vi "Material-Laser-ChangeSamplingRate.vi"(8 "error in (no error)":errorcluster, 11 "Material-RunTest in":refnum<class "Material-RunTest.lvclass">) -> (0 "error out":errorcluster, 2 "Rate updated?":bool, 3 "Material-RunTest out":refnum<class "Material-RunTest.lvclass">)   [LabVIEW 2013, in "Material-RunTest.lvclass"]
uses:
  Material-RunTest.lvclass
  Material-RunTest.lvclass/Material-RunTest.ctl
  <instrlib>/Keyence LK-G5000/Public/enum/LKIF_SamplingRate.ctl
  <instrlib>/Keyence LK-G5000/Keyence LK-G5000.lvlib
  <vilib>/addons/_LabVIEW Style Book/Utilities/Style Book Utilities.lvlib
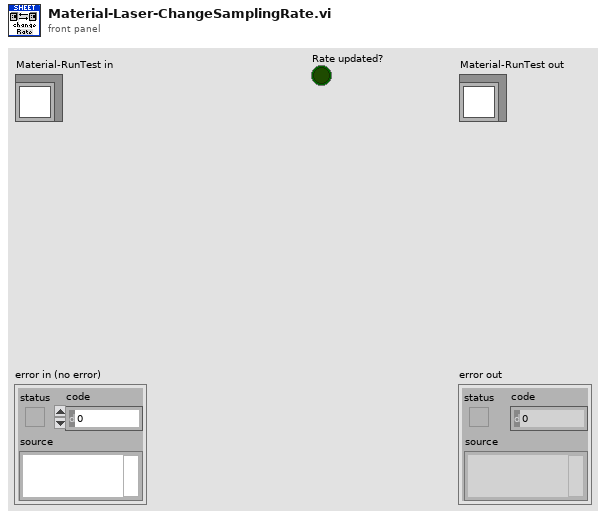
[diagram p1: front panel]
types:
  T1 = typedef "Keyence LK-G5000.lvlib/LKIF_SamplingRate.ctl" = enum16{"2.55uSEC", "5uSEC", "10uSEC", "20uSEC", "50uSEC", "100uSEC", "200uSEC", "500uSEC", "1mSEC"}
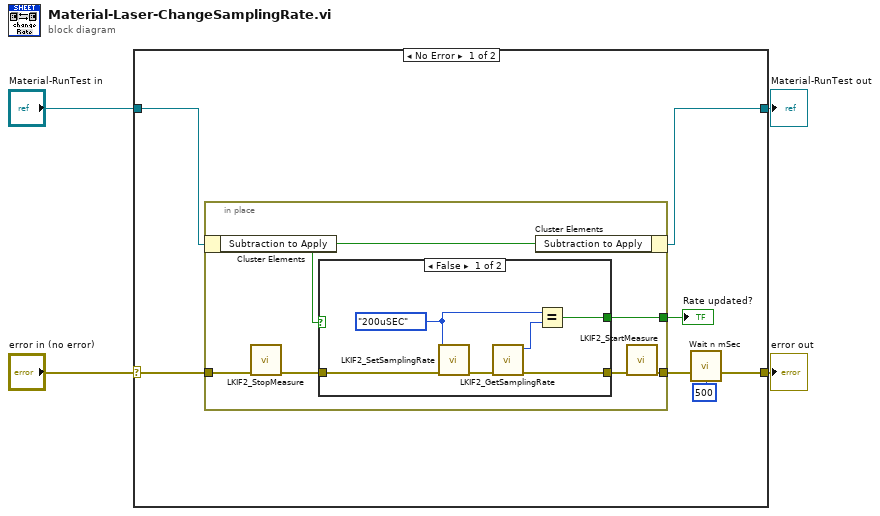
[diagram p0: block diagram]
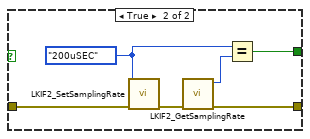
[diagram p2: hidden frame]
diagram:
  n1 = case shown="No Error" "error in (no error)" {
    selector: "error in (no error)" -> [w10 w31]
    tunnel: [w6 w31] -> w3
    tunnel: [w9 w30] -> w1
    tunnel: "Material-RunTest in" -> [w11 w30]
    frame No Error {
      n2 = in-place {
        in-place-border: w10 -> [w17]
        in-place-border: [w14] -> w7
        in-place-border: [w12] -> w8
        n3 = in-place-cluster #1(w11) -> ("Subtraction to Apply"=w13:bool)
        n4 = call <instrlib>:"LKIF2_StopMeasure.vi"("error in (no error)"=w17) -> ("error out"=w16:errorcluster)  [unwired: 10 in]
        n5 = case shown="False" w13 {
          tunnel: w16 -> [w23 w29]
          tunnel: [w21 w26] -> w15
          tunnel: [w18 w24] -> w12
          frame False {
            w20 = LKIF_SamplingRate."200uSEC" ("Sampling Rate")
            n6 = call <instrlib>:"LKIF2_SetSamplingRate.vi"("error in (no error)"=w23, "Sampling Rate"=w20) -> ("error out"=w22:errorcluster)  [unwired: 9 in]
            n7 = call <instrlib>:"LKIF2_GetSamplingRate.vi"("error in"=w22) -> ("error out"=w21:errorcluster, "Sampling Rate"=w19:T1)  [unwired: 9 in]
            n8 = Equal?(x=w20, y=w19) -> (x = y?=w18:bool)
          }
          frame True {
            w25 = LKIF_SamplingRate."200uSEC" ("Sampling Rate")
            n9 = call <instrlib>:"LKIF2_SetSamplingRate.vi"("error in (no error)"=w29, "Sampling Rate"=w25) -> ("error out"=w27:errorcluster)  [unwired: 9 in]
            n10 = call <instrlib>:"LKIF2_GetSamplingRate.vi"("error in"=w27) -> ("error out"=w26:errorcluster, "Sampling Rate"=w28:T1)  [unwired: 9 in]
            n11 = Equal?(x=w25, y=w28) -> (x = y?=w24:bool)
          }
        }
        n12 = in-place-cluster #1("Subtraction to Apply"=w13) -> (w9:refnum<class "Material-RunTest.lvclass">)
        n13 = call <instrlib>:"LKIF2_StartMeasure.vi"("error in (no error)"=w15) -> ("error out"=w14:errorcluster)  [unwired: 10 in]
      }
      "Rate updated?" <- w8
      n14 = call <vilib>:"Wait n mSec.vi"("error in (no error)"=w7, "Milliseconds to Wait (500)"=u32 500) -> ("error out"=w6:errorcluster)  [unwired: 13 in]
    }
    frame Error {
    }
  }
  "error out" <- w3
  "Material-RunTest out" <- w1
